vi "PasteCSV.vi"(6 "Variant in":variant, 7 "Shift Pressed?":bool, 8 "error in (no error)":errorcluster, 10 "QD Combo Box Ref":refnum<vi>, 11 "QD Launch VI Ref":refnum<vi>) -> (0 "error out":errorcluster, 4 "Variant out":variant)   [LabVIEW 2018]
doc: "takes CSV data in the clipboard and pastes it into multicolumn listboxes, tables, 2D arrays (controls and constants).\n\nShift key removes the top row of the data in the clipboard (eg header info) and if possible pastes it into mclistbox / table column headers (or just leaves it out of numeric 2d arrays)\n\nBrian Bean\nSobosoft LLC.\n\nDefault Shortcut - [Q]"
panel:
  in  "Undo Name":string="Change to Array or Element"
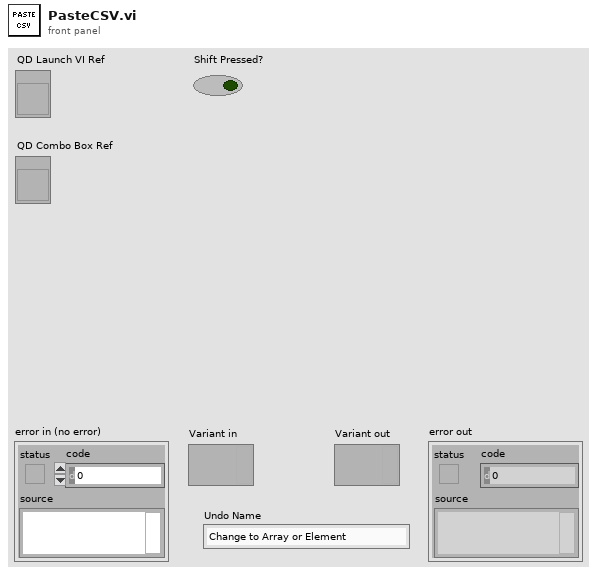
[diagram p1: front panel]
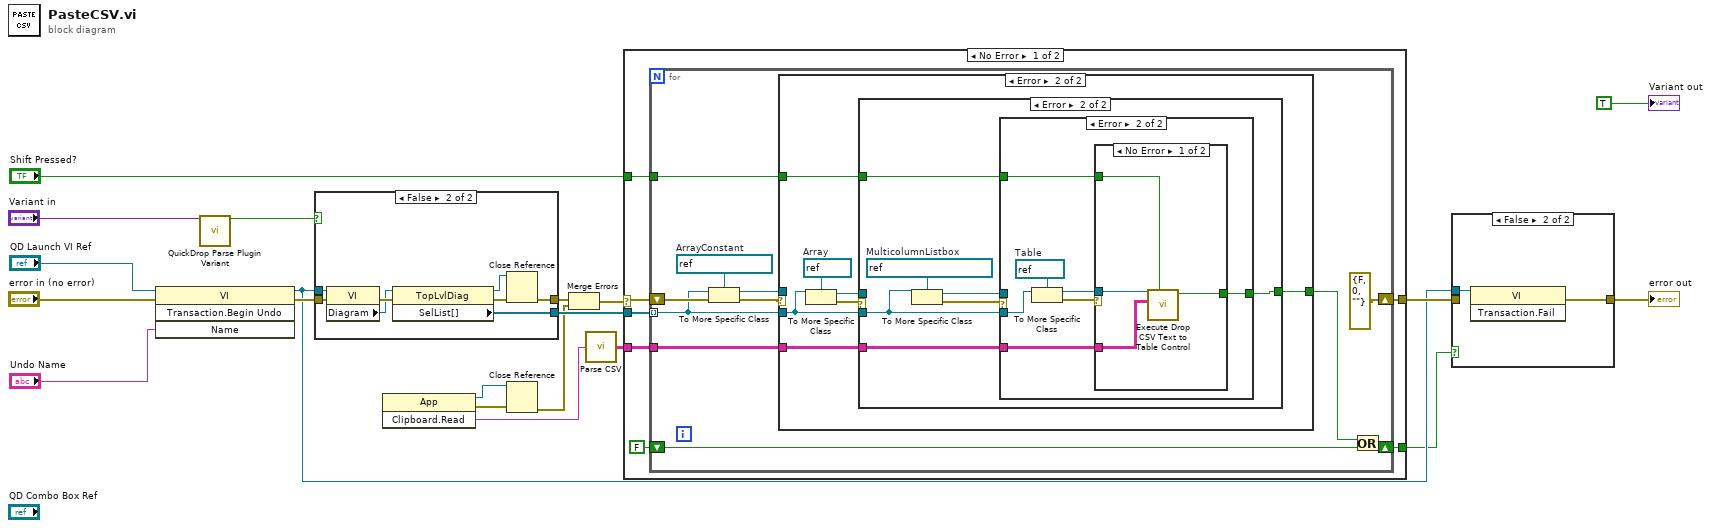
[diagram p0: block diagram]
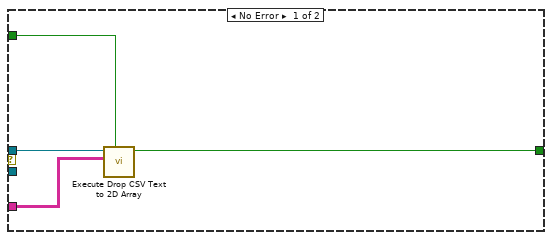
[diagram p2: hidden frame]
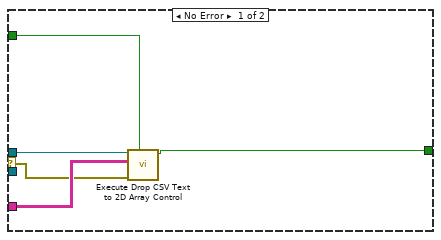
[diagram p3: hidden frame]
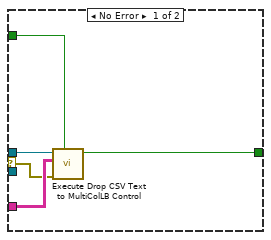
[diagram p4: hidden frame]
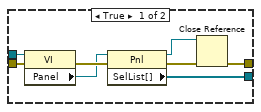
[diagram p7: hidden frame]
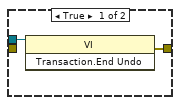
[diagram p8: hidden frame]
diagram:
  n1 = invoke class="VI" method="Transaction.Begin Undo"(reference="QD Launch VI Ref", error in="error in (no error)", "Name"="Undo Name") -> (reference out=w13:refnum<vi>, error out=w15:errorcluster)  [unwired: 1 in, 2 out]
  n2 = call <vilib>:"QuickDrop Parse Plugin Variant.vi"("QDKS Variant in"="Variant in") -> ("QD Launch VI Panel?"=w10:bool)  [unwired: 12 in, 2 out]
  n3 = case shown="False" w10 {
    tunnel: w15 -> [w28 w36]
    tunnel: w13 -> [w27 w35]
    tunnel: [w22 w30] -> w4
    tunnel: [w21 w29] -> w11
    frame True {
      n4 = property class="VI"(reference=w27, error in=w28) -> (error out=w26:errorcluster, "Panel"=w25:refnum<vi>)  [unwired: 1 out]
      n5 = property class="Pnl"(reference=w25, error in=w26) -> (reference out=w23:refnum<vi>, error out=w24:errorcluster, "SelList[]"=w21:refnum<vi>[])
      n6 = Close Reference(reference=w23, error in (no error)=w24) -> (error out=w22:errorcluster)
    }
    frame False {
      n7 = property class="VI"(reference=w35, error in=w36) -> (error out=w34:errorcluster, "Diagram"=w33:refnum<vi>)  [unwired: 1 out]
      n8 = property class="TopLvlDiag"(reference=w33, error in=w34) -> (reference out=w31:refnum<vi>, error out=w32:errorcluster, "SelList[]"=w29:refnum<vi>[])
      n9 = Close Reference(reference=w31, error in (no error)=w32) -> (error out=w30:errorcluster)
    }
  }
  n10 = invoke class="App" method="Clipboard.Read"() -> (reference out=w6:refnum<vi>, error out=w7:errorcluster, "Read Clipbrd"=w2:string)  [unwired: 3 in]
  n11 = Close Reference(reference=w6, error in (no error)=w7) -> (error out=w5:errorcluster)
  n12 = Merge Errors(w4, w5) -> (w3:errorcluster)
  n13 = call "Parse CSV.vi"("CSV String"=w2) -> ("2D Array"=w1:string[][])  [unwired: 4 in]
  n14 = case shown="No Error" w3 {
    selector: w3 -> [w38 w94]
    tunnel: [w43 w94] -> w14
    tunnel: [w41 _] -> w12
    tunnel: w11 -> [w40 _]
    tunnel: "Shift Pressed?" -> [w39 _]
    tunnel: w1 -> [w37 _]
    frame No Error {
      n15 = for {
        shift-right: [errorcluster {"status"=FALSE, "code"=0, "source"=""} ("error out")] -> w43
        shift-left: w38 -> [w52]
        shift-right: [w53] -> w41
        shift-left: FALSE -> [w54]
        tunnel: w40 -> [w46] mode=indexing
        tunnel: w39 -> [w45]
        tunnel: w37 -> [w44]
        w49 = refnum<vi> refnum  # ArrayConstant
        n16 = To More Specific Class(target class=w49, reference=w46, error in=w52) -> (specific class reference=w48:refnum<vi>, error out=w47:errorcluster)
        n17 = case shown="Error" w47 {
          tunnel: [w58 w65] -> w51
          tunnel: w48 -> [w57 _]
          tunnel: w46 -> [_ w60]
          tunnel: w45 -> [w56 w62]
          tunnel: w44 -> [w55 w59]
          frame No Error {
            n18 = call "Execute Drop CSV Text to 2D Array.vi"("Shihft (F)"=w56, "2D Array"=w55, "Const"=w57) -> ("success?"=w58:bool)  [unwired: 8 in]
          }
          frame Error {
            w64 = refnum<vi> refnum  # Array
            n19 = To More Specific Class(target class=w64, reference=w60) -> (specific class reference=w63:refnum<vi>, error out=w61:errorcluster)  [unwired: 1 in]
            n20 = case shown="Error" w61 {
              selector: w61 -> [w66 _]
              tunnel: [w70 w72] -> w65
              tunnel: w63 -> [w69 _]
              tunnel: w62 -> [w68 w75]
              tunnel: w60 -> [_ w74]
              tunnel: w59 -> [w67 w71]
              frame No Error {
                n21 = call "Execute Drop CSV Text to 2D Array Control.vi"("Shift (F)"=w68, "Error In"=w66, "Table Control"=w67, "Control"=w69) -> ("success?"=w70:bool)  [unwired: 7 in]
              }
              frame Error {
                w77 = refnum<vi> refnum  # MulticolumnListbox
                n22 = To More Specific Class(target class=w77, reference=w74) -> (specific class reference=w76:refnum<vi>, error out=w73:errorcluster)  [unwired: 1 in]
                n23 = case shown="Error" w73 {
                  selector: w73 -> [w78 _]
                  tunnel: w76 -> [w82 _]
                  tunnel: w75 -> [w81 w84]
                  tunnel: w74 -> [_ w88]
                  tunnel: [w80 w85] -> w72
                  tunnel: w71 -> [w79 w83]
                  frame No Error {
                    n24 = call "Execute Drop CSV Text to MultiColLB Control.vi"("Shift (F)"=w81, "error in"=w78, "2D Array"=w79, "Control"=w82) -> ("success?"=w80:bool)  [unwired: 7 in]
                  }
                  frame Error {
                    w89 = refnum<vi> refnum  # Table
                    n25 = To More Specific Class(target class=w89, reference=w88) -> (specific class reference=w86:refnum<vi>, error out=w87:errorcluster)  [unwired: 1 in]
                    n26 = case shown="No Error" w87 {
                      tunnel: w86 -> [w93 _]
                      tunnel: [w92 _] -> w85
                      tunnel: w84 -> [w91 _]
                      tunnel: w83 -> [w90 _]
                      frame No Error {
                        n27 = call "Execute Drop CSV Text to Table Control.vi"("Shihft (F)"=w91, "2D Array"=w90, "Control"=w93) -> ("success?"=w92:bool)  [unwired: 8 in]
                      }
                      frame Error {
                      }
                    }
                  }
                }
              }
            }
          }
        }
        n28 = Or(x=w51, y=w54) -> (x .or. y?=w53:bool)
      }
    }
    frame Error {
    }
  }
  n29 = case shown="False" w12 {
    tunnel: w13 -> [w95 w97]
    tunnel: [w96 w98] -> w19
    tunnel: w14 -> [_ _]
    frame True {
      n30 = invoke class="VI" method="Transaction.End Undo"(reference=w95) -> (error out=w96:errorcluster)  [unwired: 2 in, 2 out]
    }
    frame False {
      n31 = invoke class="VI" method="Transaction.Fail"(reference=w97) -> (error out=w98:errorcluster)  [unwired: 2 in, 2 out]
    }
  }
  "error out" <- w19
  "Variant out" <- TRUE
